vi "HAB Climber.vi"() -> ()   [LabVIEW 2018]
uses:
  <vilib>/Rock Robotics/SystemInterfaces/DIO/FPGA_DIOChannel.ctl
  <vilib>/Rock Robotics/WPI/ThirdParty/Phoenix-LabVIEW/Motor Controller/Controls/CTRE_Phoenix_MotorControl_ControlMode.ctl
  <vilib>/Rock Robotics/WPI/Switch/WPI_SwitchOpenLimit.vi
  Times/Times Global.vi
  HAB Climber Global.vi
  Robot Information/Robot Information Global.vi
panel:
  out "HAB Lock":bool
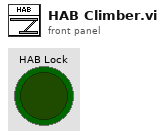
[diagram p1: front panel]
types:
  T1 = typedef "FPGA_DIOChannel.ctl" = enum8{"DIO 0", "DIO 1", "DIO 2", "DIO 3", "DIO 4", "DIO 5", "DIO 6", "DIO 7", "DIO 8", "DIO 9", "DIO MXP 0", "DIO MXP 1", "DIO MXP 2", "DIO MXP 3", "DIO MXP 4", "DIO MXP 5", "DIO MXP 6", "DIO MXP 7", "DIO MXP 8", "DIO MXP 9", "DIO MXP 10", "DIO MXP 11", "DIO MXP 12", "DIO MXP 13", "DIO MXP 14", "DIO MXP 15", "SPI Port CS1", "SPI Port CS2", "SPI Port CS3", "SPI Port MISO", "SPI Port MOSI", "Invalid"}
  T2 = typedef "WPI_SwitchDevRef.ctl" = cluster{"DevStatus":errorcluster, "DIO Channel":T1, "CntIndex":T3, "Normally Closed":bool}
  T3 = typedef "FPGA_CounterCtrSystemIndex.ctl" = enum8{"Ctr 0", "Ctr 1", "Ctr 2", "Ctr 3", "Ctr 4", "Ctr 5", "Ctr 6", "Ctr 7", "Invalid"}
  T4 = typedef "WPI_MotorControlDeviceRef.ctl" = cluster{"DeviceStatus":errorcluster, "Type":T5, "PWM":cluster{"PWM Channel":T6, "DeadBand":T7}, "CAN":cluster{"Device Number":u8, "SetOutput VI Ref":variant, "GetOutput VI Ref":variant, "Enable VI Ref":variant, "Disable VI Ref":variant, "Data":variant}, "Invert":bool, "DIO PWM":cluster{"PWM \"Enable\" Channel":T6, "DIOChannel":T1, "PWM Rate":dbl}}
  T5 = typedef "WPI_MotorControlType.ctl" = enum16{"PWM", "CAN", "DIO PWM"}
  T6 = typedef "FPGA_DIOPWMChannel.ctl" = enum8{"PWM 0", "PWM 1", "PWM 2", "PWM 3", "PWM 4", "PWM 5", "PWM 6", "PWM 7", "PWM 8", "PWM 9", "PWM MXP 0", "PWM MXP 1", "PWM MXP 2", "PWM MXP 3", "PWM MXP 4", "PWM MXP 5", "PWM MXP 6", "PWM MXP 7", "PWM MXP 8", "PWM MXP 9", "Invalid"}
  T7 = typedef "WPI_PWMDeadband.ctl" = cluster{"Name":string, "maxPositivePwm":i32, "minPositivePwm":i32, "centerPwm":i32, "maxNegativePwm":i32, "minNegativePwm":i32, "angularRange":u16}
  T8 = typedef "CTRE_Phoenix_MotorControl_ControlMode.ctl" = u16
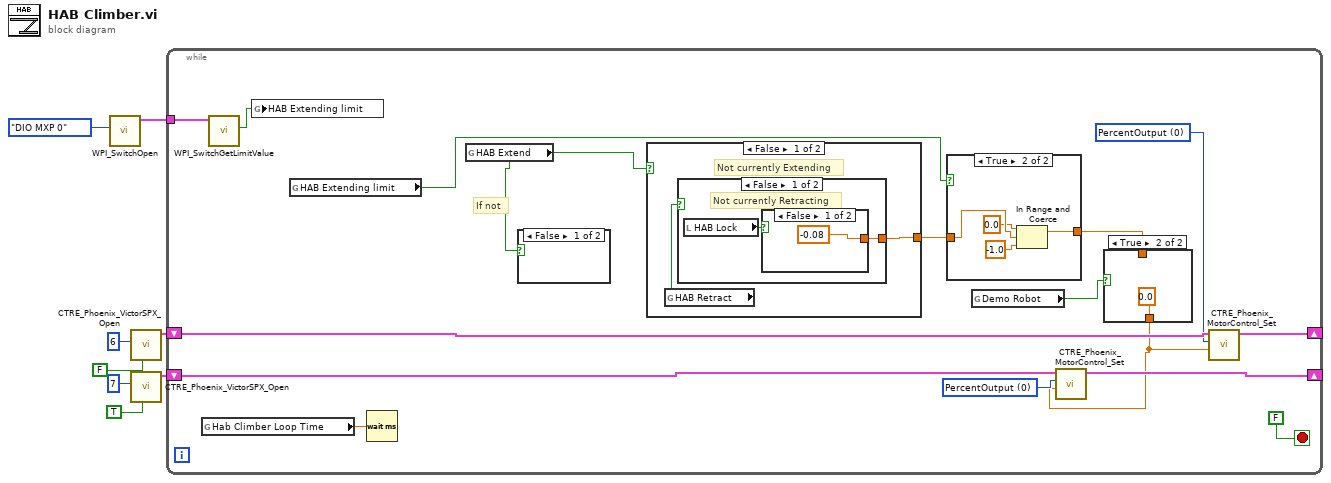
[diagram p0: block diagram]
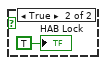
[diagram p3: hidden frame]
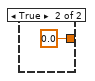
[diagram p4: hidden frame]
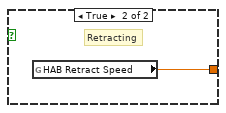
[diagram p5: hidden frame]
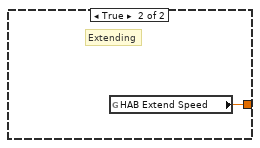
[diagram p6: hidden frame]
diagram:
  n1 = call-poly <vilib>:"WPI_SwitchOpen.vi"("DIO Channel"=FPGA_DIOChannel."DIO MXP 0") -> ("SwitchDevRef"=w3:T2)  [unwired: 9 in, 1 out]
  n2 = call <vilib>:"CTRE_Phoenix_VictorSPX_Open.vi"("Invert"=FALSE, "Device Number"=u8 6) -> ("CAN Talon SRX Ref"=w8:T4)  [unwired: 8 in, 1 out]
  n3 = call <vilib>:"CTRE_Phoenix_VictorSPX_Open.vi"("Invert"=TRUE, "Device Number"=u8 7) -> ("CAN Talon SRX Ref"=w6:T4)  [unwired: 8 in, 1 out]
  n4 = while {
    shift-right: [w20] -> _
    shift-left: w8 -> [w22]
    shift-right: [w19] -> _
    shift-left: w6 -> [w21]
    tunnel: w3 -> [w18]
    stop <- FALSE stop-if-true
    w13 = T8 0 items=["PercentOutput"=0, "Position"=1, "Velocity"=2, "Current"=3, "Follower"=5, "MotionProfile"=6, "MotionMagic"=7, "MotionProfileArc"=10, "Disabled"=15] ("Control Mode")
    w14 = T8 0 items=["PercentOutput"=0, "Position"=1, "Velocity"=2, "Current"=3, "Follower"=5, "MotionProfile"=6, "MotionMagic"=7, "MotionProfileArc"=10, "Disabled"=15] ("Control Mode")
    # "If not"
    n5 = global read "Times Global.vi" "Hab Climber Loop Time"() -> (w24:dbl)
    n6 = call <vilib>:"WPI_SwitchGetLimitValue.vi"("SwitchDevRef"=w18) -> ("Switch Pressed"=w16:bool)  [unwired: 8 in, 2 out]
    n7 = global write "HAB Climber Global.vi" "HAB Extending limit"(w16) -> ()
    n8 = global read "HAB Climber Global.vi" "HAB Extending limit"() -> (w17:bool)
    n9 = Wait (ms)(milliseconds to wait=w24) -> ()  [unwired: 1 out]
    n10 = global read "HAB Climber Global.vi" "HAB Extend"() -> (w12:bool)
    n11 = case shown="False" w12 {
      frame False {
      }
      frame True {
        "HAB Lock" <- TRUE ("HAB Lock")
      }
    }
    n12 = case shown="False" w12 {
      tunnel: [w29 w35] -> w15
      frame False {
        # "Not currently Extending"
        n13 = global read "HAB Climber Global.vi" "HAB Retract"() -> (w28:bool)
        n14 = case shown="False" w28 {
          tunnel: [w31 w34] -> w29
          frame False {
            # "Not currently Retracting"
            n15 = local read "HAB Lock"() -> (w30:bool)
            n16 = case shown="False" w30 {
              tunnel: [-0.08 0.0] -> w31
              frame False {
              }
              frame True {
              }
            }
          }
          frame True {
            # "Retracting"
            n17 = global read "HAB Climber Global.vi" "HAB Retract Speed"() -> (w34:dbl)
          }
        }
      }
      frame True {
        # "Extending"
        n18 = global read "HAB Climber Global.vi" "HAB Extend Speed"() -> (w35:dbl)
      }
    }
    n19 = case shown="True" w17 {
      tunnel: w15 -> [w36 w40]
      tunnel: [w36 w37] -> w10
      frame False {
      }
      frame True {
        n20 = In Range and Coerce(upper limit=0.0, x=w40, lower limit=-1.0) -> (coerced(x)=w37:dbl)  [unwired: 1 out]
      }
    }
    n21 = global read "Robot Information Global.vi" "Demo Robot"() -> (w9:bool)
    n22 = case shown="True" w9 {
      tunnel: [w25 0.0 ("upper limit")] -> w11
      tunnel: w10 -> [w25 _]
      frame False {
      }
      frame True {
      }
    }
    n23 = call <vilib>:"CTRE_Phoenix_MotorControl_Set.vi"("Output"=w11, "Control Mode"=w13, "PhoenixMotorControlDevRef"=w21) -> ("PhoenixMotorControlDevRef"=w19:T4)  [unwired: 7 in, 1 out]
    n24 = call <vilib>:"CTRE_Phoenix_MotorControl_Set.vi"("Output"=w11, "Control Mode"=w14, "PhoenixMotorControlDevRef"=w22) -> ("PhoenixMotorControlDevRef"=w20:T4)  [unwired: 7 in, 1 out]
  }
